vi "Boonton7200_Configure_CV.vi"(8 "Error In":errorcluster, 9 "Capacitance Range":T1, 10 "Start Bias":dbl, 11 "GPIB Address Sting":string) -> (0 "Error Out":errorcluster)   [LabVIEW 2015, in "Boonton7200.lvlib"]
uses:
  Boonton7200.lvlib
  Boonton7200_Special_Function_Codes.ctl
  Boonton7200_IEEE-488_Bus_Mnemonics.ctl
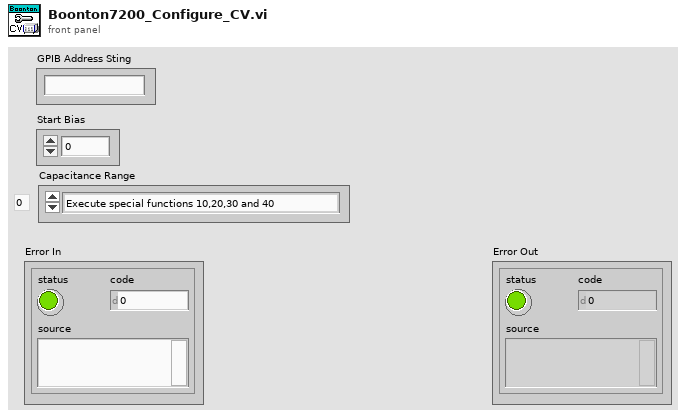
[diagram p1: front panel]
types:
  T1 = typedef "Boonton7200_Special_Function_Codes.ctl" = enum16{"Execute special functions 10,20,30 and 40", "Test Level display and entry", "Capacitance Standard display and entry", "Conductance Standard dispaly and entry", "Capacitance Low Limit display and entry", "Capacitance High Limit dispaly and entry", "IEEE-488 Bus Address display and entry", "End-of-string charecter display and selection", "Capacitance uncertainty display", "Conductance uncertainty dispaly", "Automatic selection(Measurement Ranging Functions)", "Hold current measurement range", "Set and hold 2.000 pF / 2.00 uS range", "Set and hold 20.00 pF / 20.0 uS range", "Set and hold 200.0 pF / 200 uS range", "Set and holde 2000 pF / 2000 uS range", "16 - Not Defined", "17 - Not Defined", "18 - Not Defined", "19 - Not Defined", "Automatic selection(Internal Bias Ranging Functions)", "Hold current bias range", "Set and hold 20.000 V range", "Set and Hold 100.00 V range", "24 - Not Defined", "25 - Not Defined", "26 - Not Defined", "27 - Not Defined", "28 - Not Defined", "29 - Not Defined", "30 Automatic selection(Measurement Filter Functions)", "Filter length = 1 measurement, no average", "Filter length = 2 measurement", "Filter length = 5 measurement", "Filter length = 10 measurement", "Filter length = 20 measurement", "Filter length = 50 measurement", "Filter length = 100 measurement", "Filter length = 200 measurement", "Filter length = 500 measurement", "Normal operation, free-run dispaly(Sercvice Request Functions)", "Disable SRQ interrupt", "Enable SRQ interrupt", "Set SRQ mask when an error occurs", "Set SRQ mask and update dispaly when measurement filter is complete", "Set SRQ mask when capacitance measurement is within the high and low limit settings", "Set SRQ mask when capacitance measurement exceeds the high or low limit settings", "Set SRQ mask when zero or calibration is complete", "Set SRQ mask when sweep is complete", "49 - Not Defined", "Calibrate detector offset(Automatic Calibration and Test Functions)", "Calibrate external bias offset", "Calibrate internal bias offset", "Calibrate full-scale capacitance", "Calibrate conductance phase", "Display internal temperature", "Display amplitude error due to temperature influence", "Display phase error due to temperature influence", "Initialize instrument and erase all program locations", "Initalize software calibration variables"}
  T2 = typedef "Boonton7200_IEEE-488_Bus_Mnemonics.ctl" = string
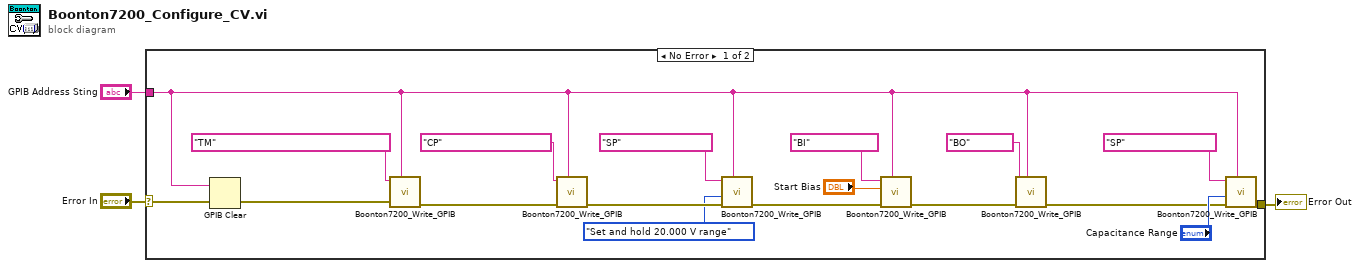
[diagram p0: block diagram]
diagram:
  n1 = case shown="No Error" "Error In" {
    selector: "Error In" -> [w12 w22]
    tunnel: [w11 w22] -> w2
    tunnel: "GPIB Address Sting" -> [w5 _]
    frame No Error {
      n2 = GPIB Clear(2:w12, 3:w5) -> (0:w7:errorcluster)  [unwired: 1 out]
      n3 = call "Boonton7200_Write_GPIB.vi"("GPIB Address String"=w5, "Error In"=w7, "IEEE-488 Bus Mnemonics"=T2 "TM") -> ("Error Out"=w6:errorcluster)  [unwired: 8 in]
      n4 = call "Boonton7200_Write_GPIB.vi"("GPIB Address String"=w5, "Error In"=w6, "IEEE-488 Bus Mnemonics"=T2 "CP") -> ("Error Out"=w20:errorcluster)  [unwired: 8 in]
      n5 = call "Boonton7200_Write_GPIB.vi"("GPIB Address String"=w5, "Error In"=w20, "Special Functions"=Boonton7200_Special_Function_Codes."Set and hold 20.000 V range", "IEEE-488 Bus Mnemonics"=T2 "SP") -> ("Error Out"=w17:errorcluster)  [unwired: 7 in]
      n6 = call "Boonton7200_Write_GPIB.vi"("GPIB Address String"=w5, "Error In"=w17, "Data Value"="Start Bias", "IEEE-488 Bus Mnemonics"=T2 "BI") -> ("Error Out"=w9:errorcluster)  [unwired: 7 in]
      n7 = call "Boonton7200_Write_GPIB.vi"("GPIB Address String"=w5, "Error In"=w9, "IEEE-488 Bus Mnemonics"=T2 "BO") -> ("Error Out"=w8:errorcluster)  [unwired: 8 in]
      n8 = call "Boonton7200_Write_GPIB.vi"("GPIB Address String"=w5, "Error In"=w8, "Special Functions"="Capacitance Range", "IEEE-488 Bus Mnemonics"=T2 "SP") -> ("Error Out"=w11:errorcluster)  [unwired: 7 in]
    }
    frame Error {
    }
  }
  "Error Out" <- w2
